vi "Object in Elevator.vi"() -> (3 "Ping Detect":bool)   [LabVIEW 2014]
uses:
  Elevator Command.ctl
  Robot Global Data.vi
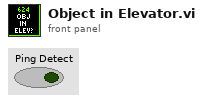
[diagram p1: front panel]
types:
  T1 = typedef "Elevator Command.ctl" = enum16{"Idle", "Load 1", "Load 2", "Load 3", "Drop Stack", "Eject Stack", "Untip Trashcan", "Load Trashcan", "HP Load", "HP Score"}
  T2 = typedef "Elevator Control Command.ctl" = cluster{"Command":T1, "Manual Motor Out":dbl, "Manual Eject Piston":bool, "Mode":T3, "Override Limits":bool, "Manual Stabilizer":bool, "Manual Finger":bool, "Store Trashcan?":bool, "Hold Low?":bool, "Idle Mode":T4, "HP Load":bool, "Unstick":bool}
  T3 = typedef "Elevator Mode.ctl" = enum16{"Manual", "Safe", "Auto"}
  T4 = typedef "Elevator Idle Mode.ctl" = enum16{"Load 1", "Load 2", "Load 3", "Load Can", "Untip Can", "Step Load", "Drop Stack"}
  T5 = typedef "Dashboard Control Data.ctl" = cluster{"Cam Exposure":dbl, "Go to angle":dbl, "Steer PID Gains":cluster{"proportional gain (Kc)":dbl, "integral time (Ti, min)":dbl, "derivative time (Td, min)":dbl}, "Steer PID output Range":cluster{"output high":dbl, "output low":dbl}, "Pressure m \nValue":dbl, "Pressure b \nValue":dbl, "Roller Command Cluster ":T6, "Elevator":T7, "Encoder Control":T9, "Auton Settings":cluster{"Drive Dist Window Size":dbl}, "Drivetrain Settings":T10, "Lance":T11}
  T6 = typedef "Roller Control.ctl" = cluster{"Intake Speed":dbl, "Turn In Speed":dbl, "Unload Speed":dbl, "Turn Out Speed":dbl, "Ping Align Tolerance":dbl, "Tote Range Threshold":dbl, "Right Pot 0":dbl, "Pot Threshold":dbl, "Left Pot 0":dbl, "Manual 0s?":bool, "Right Pot Scale":dbl, "Left Pot Scale":dbl, "0 wait time":i32, "Zero Pots":bool, "Min Elevator Height":dbl, "Eject Time":dbl, "Eject US Threshold":dbl, "Anti-Twitch Time":u32, "Ping Caring Threshold":dbl, "Pot Diff Threshold":dbl, "Pinch Sustain":u32, "Absorb Give Up Threshold":dbl, "Untip In Threshold":dbl, "Untip Grab Range":dbl, "Ultrasonic Hold Time":u32, "Landscape Absorb Time":u32, "Pot Use Wait Time":u32, "Can Turn Stop Range":dbl, "Ignore Pressure":bool, "HP Load Speed":dbl}
  T7 = typedef "Elevator DB Control.ctl" = cluster{"PID Output Range":cluster{"output high":dbl, "output low":dbl}, "PID gains":cluster{"proportional gain (Kc)":dbl, "integral time (Ti, min)":dbl, "derivative time (Td, min)":dbl}, "Height Tolerance":sgl, " Encoder Constant":dbl, "Safe Mode Max Speed":sgl, "Eject Time":sgl, "Zeroing Speed":sgl, "Presets":T8, "Ping Detect Threshold":sgl, "Trashcan Detect Threshold":sgl, "Zero Filter Time":dbl, "Stabilizer Open Time":dbl, "Zero Creep Speed":dbl, "Max Current":dbl, "Current Trip Time":dbl, "Abort Pitch":dbl, "Finger m":dbl, "Finger b":dbl, "Finger max ":dbl, "Finger Stabilizer":dbl, "Finger Store":dbl, "Finger Stop Store":dbl, "Stabilizer Close Time":dbl, "HP Finger Store":dbl, "HP Finger Stop Store":dbl, "Finger min":dbl, "Unstick gain":dbl, "Roller Wait":dbl}
  T8 = typedef "Elevator Presets.ctl" = cluster{"Pickup 2 w/ Tote":sgl, "Pickup 2 w/ Trashcan":sgl, "Pickup 3 w/ Tote":sgl, "Pickup 3 w/ Trashcan":sgl, "Bottom":sgl, "Pickup 1 w/ Tote":sgl, "Pickup Trashcan":sgl, "Pickup 1 w/ Trashcan":sgl, "Eject":sgl, "Hold Low":sgl, "Step add height":sgl, "Untip Lift":dbl, "Drop Stack":dbl, "HP Load Hold":dbl, "HP Load Drop":dbl, "HP Load Finger":dbl, "HP Load Hold Can":dbl, "Store can max":dbl, "HP Drag Score":dbl, "HP Store can max":dbl, "HP Drag Finish":dbl, "HP Carry min":dbl, "HP Finger Anti-Crash":dbl, "Finger trashcan avoid":dbl}
  T9 = typedef "Encoder Control.ctl" = cluster{"Left Tick Constant":dbl, "Right Tick Constant":dbl, "Center Tick Constant":dbl, "Reset?":bool, "Y Dist":cluster{"PID gains":cluster{"proportional gain (Kc)":dbl, "integral time (Ti, min)":dbl, "derivative time (Td, min)":dbl}}, "X Dist":cluster{"PID gains":cluster{"proportional gain (Kc)":dbl, "integral time (Ti, min)":dbl, "derivative time (Td, min)":dbl}}, "Y Stop Thresh":dbl, "Y Stop Speed":dbl, "X Stop Thresh":dbl, "X Stop Speed":dbl}
  T10 = typedef "Drivetrain Settings.ctl" = cluster{"Gyro Tolerance":sgl, "Strafe Correct max steer":sgl, "Strafe Timer Wait":sgl, "Throttle Ramp (ms)":sgl, "Strafe Ramp (ms)":sgl, "Angular rate compensation":bool, "Throttle to Rate Scale":sgl, "Rate compensation gain":sgl, "Creep Steer":sgl, "Creep Throttle":sgl}
  T11 = typedef "Pike DB Controls.ctl" = cluster{"Down Speed":dbl, "Up Speed":dbl, "Max Down Time":dbl, "Max Up Time":dbl, "Current Limit":dbl}
  T12 = typedef "Ultrasonic Indicators.ctl" = cluster{"Left Distance":dbl, "Right Distance":dbl, "Center Distance":dbl, "Left Distance Unfilter":dbl, "Right Distance Unfilter":dbl, "Center Distance Unfilter":dbl}
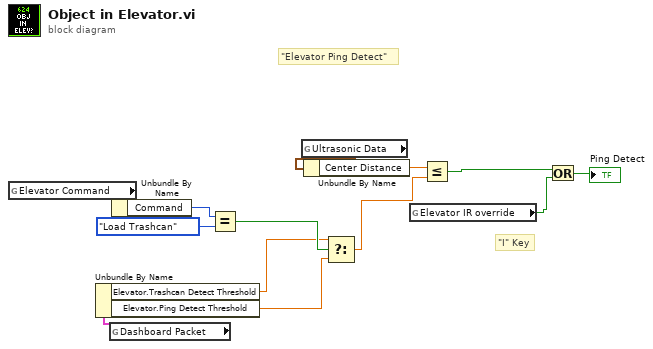
[diagram p0: block diagram]
diagram:
  # "\"I\" Key"
  # "\"Elevator Ping Detect\""
  n1 = global read "Robot Global Data.vi" "Elevator Command"() -> (w7:T2)
  n2 = global read "Robot Global Data.vi" "Dashboard Packet"() -> (w11:T5)
  n3 = Unbundle By Name(w11) -> ("Elevator.Trashcan Detect Threshold"=w2:sgl, "Elevator.Ping Detect Threshold"=w3:sgl)
  n4 = Unbundle By Name(w7) -> ("Command"=w6:T1)
  n5 = Equal?(x=w6, y=Elevator_Command."Load Trashcan") -> (x = y?=w4:bool)
  n6 = global read "Robot Global Data.vi" "Ultrasonic Data"() -> (w13:T12)
  n7 = Unbundle By Name(w13) -> ("Center Distance"=w12:dbl)
  n8 = Select(t=w2, s=w4, f=w3) -> (s? t:f=w1:sgl)
  n9 = global read "Robot Global Data.vi" "Elevator IR override"() -> (w10:bool)
  n10 = Less Or Equal?(x=w12, y=w1) -> (x <= y?=w9:bool)
  n11 = Or(x=w9, y=w10) -> (x .or. y?=→"Ping Detect":bool)
